vi "niRFUtil WFM Phase Continuous Resample (complex).vi"(0 "Waveform In":T1 {"y" format="%.2f"; "dx" format="%^.2e"; "x0" format="%^.2e"}, 1 "Initial Sample Offset (s)":dbl format="%^.3g", 2 "Allowable Sample Rate Error (ppm)":dbl=1.0 format="%^.3g", 5 "Desired Sample Rate (Hz)":dbl format="%^.3g", 9 "Waveform Quantum (4)":i32=4, 11 "error in (no error)":errorcluster, 12 "Reset? (T)":bool=TRUE, 13 "Flush Buffers? (F)":bool, 14 "Phase Continuous (T)":bool=TRUE) -> (4 "Waveform Out":T1 {"y" format="%.2f"; "dx" format="%^.2e"; "x0" format="%^.2e"}, 8 "Actual Sample Rate (Hz)":dbl format="%^.3g", 15 "error out":errorcluster)   [LabVIEW 2015, in "niRFUtil.lvlib"]
uses:
  niRFUtil.lvlib
  Includes/niRFUtil INC Complex Waveform.ctl
  Includes/niRFUtil INC Complex Array.ctl
  niRFUtil WFM Parse Waveform - Duration (complex wfm).vi
  niRFUtil WFM Concatenate Waveforms (complex wfm).vi
  Measurements/niRFUtil MEAS Waveform Statistics (complex wfm).vi
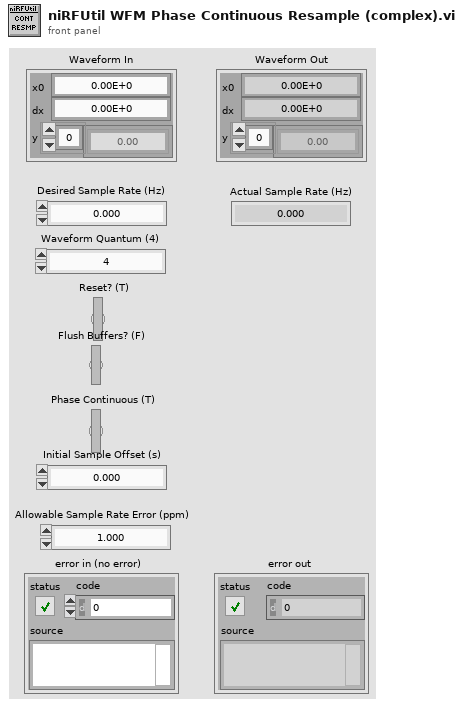
[diagram p1: front panel]
types:
  T1 = typedef "niRFUtil.lvlib/niRFUtil INC Complex Waveform.ctl" = cluster{"x0":dbl, "dx":dbl, "y":T2}
  T2 = typedef "niRFUtil.lvlib/niRFUtil INC Complex Array.ctl" = csg[]
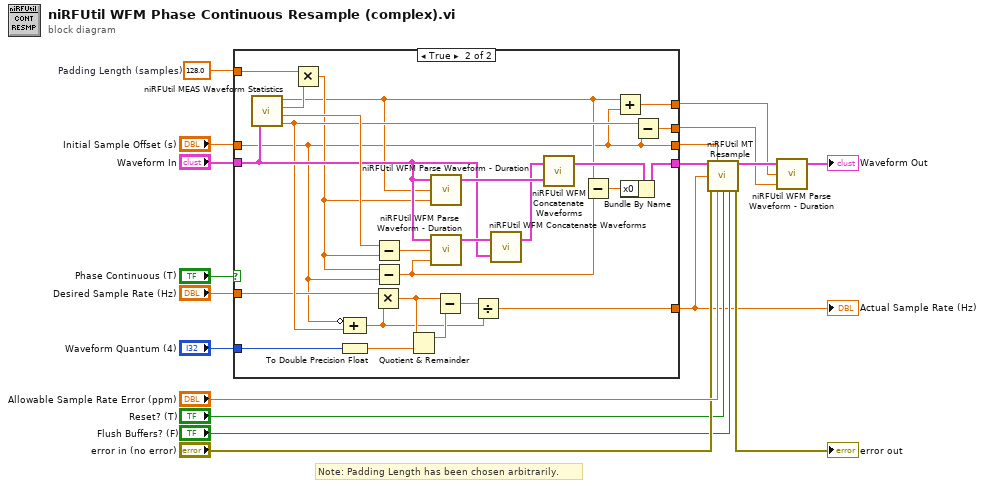
[diagram p0: block diagram]
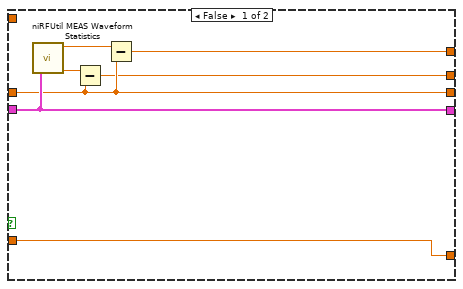
[diagram p2: hidden frame]
diagram:
  w10 = 128.0  # Padding Length (samples)
  # "Note: Padding Length has been chosen arbitrarily."
  n1 = case shown="True" "Phase Continuous (T)" {
    tunnel: [w20 w37] -> w12
    tunnel: w10 -> [_ w30]
    tunnel: "Waveform In" -> [w25 w46]
    tunnel: [w21 w27] -> w8
    tunnel: [w25 w44] -> w7
    tunnel: "Desired Sample Rate (Hz)" -> [w19 w32]
    tunnel: [w19 w40] -> w5
    tunnel: "Initial Sample Offset (s)" -> [w23 w26]
    tunnel: [w23 w26] -> w2
    tunnel: "Waveform Quantum (4)" -> [_ w39]
    frame False {
      n2 = call-poly "niRFUtil MEAS Waveform Statistics.vi"("Waveform In"=w25) -> ("Start"=w22:dbl, "Duration"=w24:dbl)  [unwired: 4 in, 2 out]
      n3 = Subtract(x=w24, y=w23) -> (x-y=w20:dbl)
      n4 = Subtract(x=w22, y=w23) -> (x-y=w21:dbl)
    }
    frame True {
      n5 = call-poly "niRFUtil MEAS Waveform Statistics.vi"("Waveform In"=w46) -> ("Start"=w28:dbl, "Interval"=w31:dbl, "End + Interval"=w51:dbl, "Duration"=w35:dbl)  [unwired: 4 in]
      n6 = Multiply(x=w30, y=w31) -> (x*y=w29:dbl)
      n7 = To Double Precision Float(number=w39) -> (double precision float=w38:dbl)
      n8 = Compound Arithmetic op=ADD(invert w26, w35) -> (w33:dbl)
      n9 = Multiply(x=w32, y=w33) -> (x*y=w43:dbl)
      n10 = Subtract(x=w51, y=w29) -> (x-y=w50:dbl)
      n11 = Subtract(x=w29, y=w26) -> (x-y=w34:dbl)
      n12 = Quotient & Remainder(x=w43, y=w38) -> (x-y*floor(x/y)=w42:dbl)  [unwired: 1 out]
      n13 = call-poly "niRFUtil WFM Parse Waveform - Duration.vi"("Duration (Inf)"=w29, "Start (-Inf)"=w28, "Waveform In"=w46) -> ("Waveform Out"=w48:T1)  [unwired: 2 in]
      n14 = call-poly "niRFUtil WFM Parse Waveform - Duration.vi"("Duration (Inf)"=w34, "Start (-Inf)"=w50, "Waveform In"=w46) -> ("Waveform Out"=w49:T1)  [unwired: 2 in]
      n15 = Subtract(x=w43, y=w42) -> (x-y=w41:dbl)
      n16 = Divide(x=w41, y=w33) -> (x/y=w40:dbl)
      n17 = call-poly "niRFUtil WFM Concatenate Waveforms.vi"("Waveform 2 In"=w46, "Waveform 1 In"=w49) -> ("Waveform Out"=w47:T1)  [unwired: 1 in]
      n18 = call-poly "niRFUtil WFM Concatenate Waveforms.vi"("Waveform 2 In"=w48, "Waveform 1 In"=w47) -> ("Waveform Out"=w45:T1)  [unwired: 1 in]
      n19 = Subtract(x=w28, y=w34) -> (x-y=w36:dbl)
      n20 = Add(x=w28, y=w26) -> (x+y=w27:dbl)
      n21 = Bundle By Name(cluster=w45, "x0"=w36) -> (w44:T1)
      n22 = Subtract(x=w35, y=w26) -> (x-y=w37:dbl)
    }
  }
  "Actual Sample Rate (Hz)" <- w5
  n23 = call "niRFUtil MT Resample.vi"("Waveform In"=w7, "initial sample offset (sec)"=w2, "desired sample rate (Hz)"=w5, "error in (no error)"="error in (no error)", "allowable sample rate error (ppm)"="Allowable Sample Rate Error (ppm)", "reset? (T)"="Reset? (T)", "flush buffers? (F)"="Flush Buffers? (F)") -> ("Waveform Out"=w13:T1, "error out"=→"error out":errorcluster)  [unwired: 7 in]
  n24 = call-poly "niRFUtil WFM Parse Waveform - Duration.vi"("Duration (Inf)"=w12, "Start (-Inf)"=w8, "Waveform In"=w13) -> ("Waveform Out"=→"Waveform Out":T1)  [unwired: 2 in]
